vi "Create Map of Parameter Names.vi"(8 "error in (no error)":errorcluster, 11 "Kasli in":refnum<class "Kasli.lvclass">) -> (0 "error out":errorcluster, 2 "Parameters Map":map{string, string[]}(c390), 3 "Kasli out":refnum<class "Kasli.lvclass">)   [LabVIEW 2020, in "Kasli Wrapper 2.0.lvlib" / "Kasli.lvclass"]
doc: "This VI reads the Build and Init.py library and retrieves the mapping of Kasli names to the list of parameters for the script"
uses:
  Kasli.lvclass
  Kasli.lvclass/Kasli.ctl
  <vilib>/regexp/Match Regular Expression.xnode
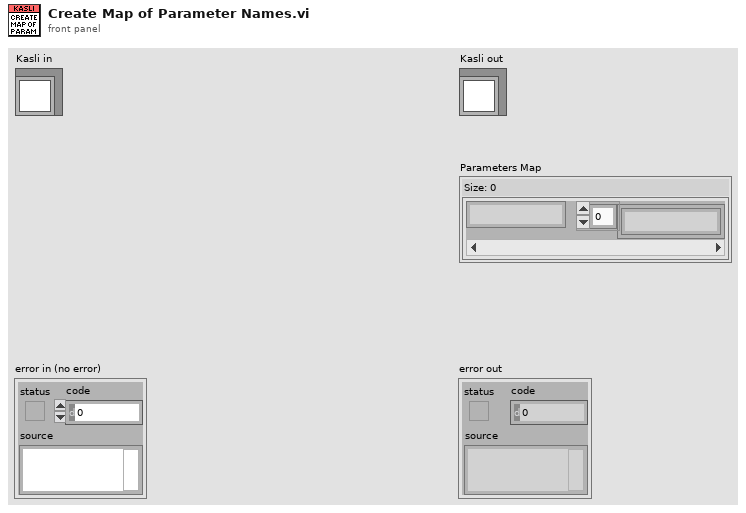
[diagram p1: front panel]
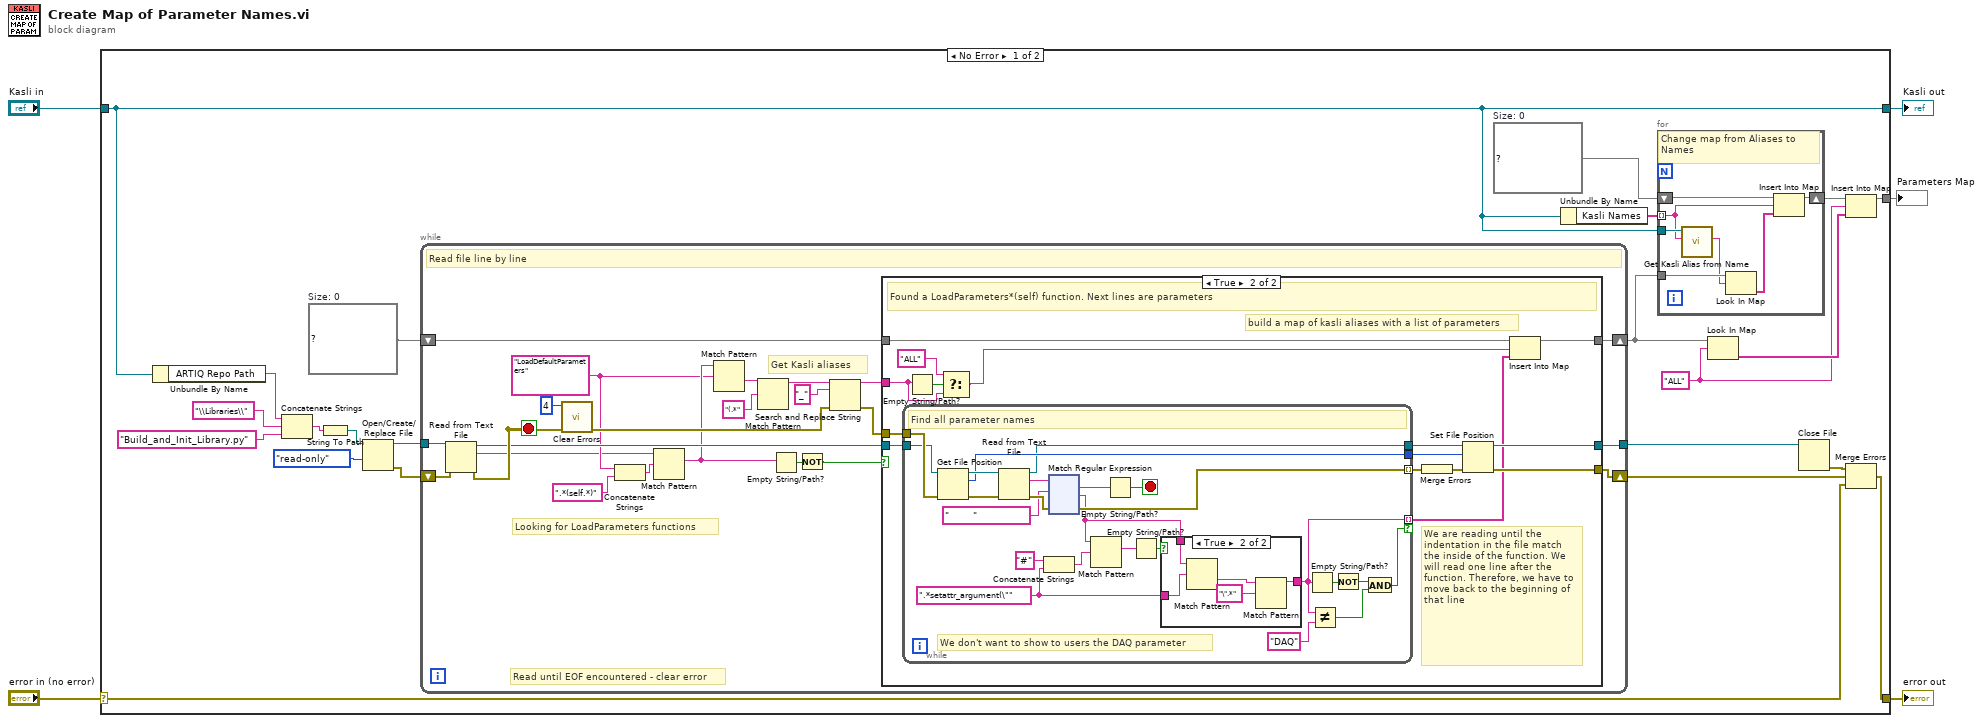
[diagram p0: block diagram]
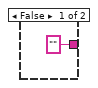
[diagram p3: hidden frame]
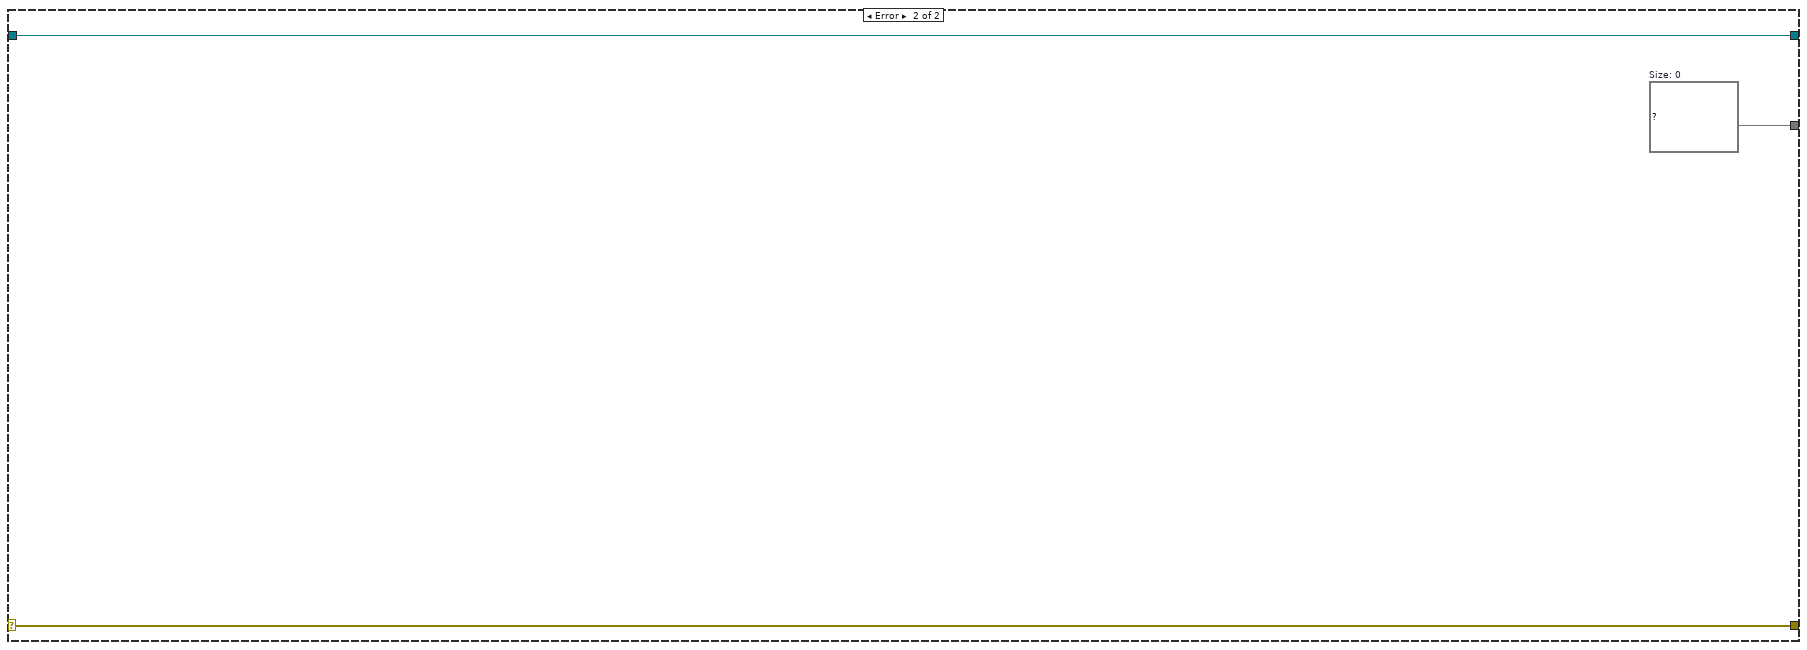
[diagram p4: hidden frame]
diagram:
  n1 = case shown="No Error" "error in (no error)" {
    selector: "error in (no error)" -> [w14 w222]
    tunnel: [w13 w222] -> w4
    tunnel: [w10 w221] -> w2
    tunnel: "Kasli in" -> [w10 w221]
    tunnel: [w9 w220] -> w1
    frame No Error {
      w6 = "ALL" ("key")
      w11 = map{string, string[]} {}  # Size: 0
      w23 = map{string, string[]} {}  # Size: 0
      n2 = Unbundle By Name(w10) -> ("ARTIQ Repo Path"=w16:string)
      n3 = Concatenate Strings(w16, "\\Libraries\\" ("string"), "Build_and_Init_Library.py") -> (w19:string)
      n4 = String To Path(string=w19) -> (path=w18:path)
      n5 = Open/Create/Replace File(file path (use dialog)=w18, access (0:read/write)=enum16{"read/write", "read-only", "write-only"}."read-only") -> (refnum out=w26:refnum<file>, error out=w15:errorcluster)  [unwired: 4 in, 1 out]
      n6 = while {
        tunnel: w26 -> [w55]
        tunnel: [w42] -> w25
        shift-right: [w46] -> w7
        shift-left: w23 -> [w47]
        shift-right: [w36] -> w22
        shift-left: w15 -> [w54]
        stop <- w56 stop-if-true
        w40 = "LoadDefaultParameters" ("regular expression")
        # "Get Kasli aliases"
        # "Looking for LoadParameters functions"
        # "Read until EOF encountered - clear error"
        # "Read file line by line"
        n7 = Read from Text File(file (use dialog)=w55, error in=w54) -> (refnum out=w44:refnum<file>, text=w35:string, error out=w56:errorcluster)  [unwired: 2 in, 1 out]
        n8 = call <vilib>:"Clear Errors.vi"("error in (no error)"=w56, "specific error code to clear (0: all)"=4) -> ("error out"=w57:errorcluster)  [unwired: 4 in, 1 out]
        n9 = Concatenate Strings(w40, ".*(self.*)" ("regular expression")) -> (w50:string)
        n10 = Match Pattern(string=w35, regular expression=w50) -> (match substring=w41:string)  [unwired: 1 in, 3 out]
        n11 = Match Pattern(string=w41, regular expression=w40) -> (after substring=w39:string)  [unwired: 1 in, 3 out]
        n12 = Match Pattern(string=w39, regular expression="(.*") -> (before substring=w37:string)  [unwired: 1 in, 3 out]
        n13 = Empty String/Path?(string/path=w41) -> (empty?=w52:bool)
        n14 = Not(x=w52) -> (.not. x?=w48:bool)
        n15 = Search and Replace String(input string=w37, search string="_", error in=w57) -> (result string=w45:string, error out=w43:errorcluster)  [unwired: 5 in, 2 out]
        n16 = case shown="True" w48 {
          tunnel: w47 -> [w60 w69]
          tunnel: [w60 w70] -> w46
          tunnel: w45 -> [_ w62]
          tunnel: w44 -> [w59 w75]
          tunnel: w43 -> [w58 w74]
          tunnel: [w59 w71] -> w42
          tunnel: [w58 w66] -> w36
          frame False {
            # "This line doesn't contain the LoadDefaultParamters function"
          }
          frame True {
            # "We are reading until the indentation in the file match the inside of the function. We will read one line after the function. Therefore, we have to move back to the beginning of that line"
            # "build a map of kasli aliases with a list of parameters"
            # "Found a LoadParameters*(self) function. Next lines are parameters"
            n17 = while {
              tunnel: w75 -> [w92]
              tunnel: w74 -> [w99]
              tunnel: [w80] -> w65 mode=indexing if=w76
              tunnel: [w87] -> w72
              tunnel: [w98] -> w67 mode=indexing
              tunnel: [w89] -> w73
              stop <- w93 stop-if-true
              w82 = ".*setattr_argument(\""
              # "We don't want to show to users the DAQ parameter"
              # "Find all parameter names"
              n18 = Get File Position(4:w99, 7:w92) -> (0:w90:errorcluster, 2:w89:i64, 3:w91:refnum<file>)
              n19 = Read from Text File(file (use dialog)=w91, error in=w90) -> (refnum out=w87:refnum<file>, text=w96:string, error out=w97:errorcluster)  [unwired: 2 in, 1 out]
              n20 = Concatenate Strings("#" ("string"), w82) -> (w83:string)
              n21 = xnode "Match Regular Expression"("input string"=w96, "regular expression"="        ", "error in"=w97) -> ("whole match"=w94:string, "after match"=w86:string, "error out"=w98:errorcluster)  [unwired: 3 in, 2 out]
              n22 = Match Pattern(string=w86, regular expression=w83) -> (match substring=w84:string)  [unwired: 1 in, 3 out]
              n23 = Empty String/Path?(string/path=w94) -> (empty?=w93:bool)
              n24 = Empty String/Path?(string/path=w84) -> (empty?=w85:bool)
              n25 = case shown="True" w85 {
                tunnel: ["" ("after match") w104] -> w80
                tunnel: w86 -> [_ w102]
                tunnel: w82 -> [_ w101]
                frame False {
                }
                frame True {
                  n26 = Match Pattern(string=w102, regular expression=w101) -> (after substring=w103:string)  [unwired: 1 in, 3 out]
                  n27 = Match Pattern(string=w103, regular expression="\".*" ("search string")) -> (before substring=w104:string)  [unwired: 1 in, 3 out]
                }
              }
              n28 = Empty String/Path?(string/path=w80) -> (empty?=w88:bool)
              n29 = Not Equal?(x=w80, y="DAQ") -> (x != y?=w77:bool)
              n30 = Not(x=w88) -> (.not. x?=w78:bool)
              n31 = And(x=w78, y=w77) -> (x .and. y?=w76:bool)
            }
            n32 = Empty String/Path?(string/path=w62) -> (empty?=w64:bool)
            n33 = Select(t="ALL", s=w64, f=w62) -> (s? t:f=w63:string)
            n34 = Merge Errors(w67) -> (w68:errorcluster)
            n35 = Set File Position(offset (in bytes) (0)=w73, refnum=w72, error in=w68) -> (refnum out=w71:refnum<file>, error out=w66:errorcluster)  [unwired: 1 in]
            n36 = Insert Into Map(map in=w69, key=w63, value=w65) -> (map out=w70:map{string, string[]})  [unwired: 2 out]
          }
        }
      }
      n37 = Unbundle By Name(w10) -> ("Kasli Names"=w12:string[])
      n38 = for {
        tunnel: w12 -> [w30] mode=indexing
        shift-right: [w33] -> w8
        shift-left: w11 -> [w34]
        tunnel: w7 -> [w32]
        tunnel: w10 -> [w31]
        # "Change map from Aliases to Names"
        n39 = call-dynamic "Get Kasli Alias from Name.vi"("Kasli Name"=w30, "Kasli in"=w31) -> ("Kasli Alias"=w29:string)  [unwired: 7 in, 2 out]
        n40 = Look In Map(map=w32, key=w29) -> (value=w28:string[])  [unwired: 1 in, 1 out]
        n41 = Insert Into Map(map in=w34, key=w30, value=w28) -> (map out=w33:map{string, string[]})  [unwired: 2 out]
      }
      n42 = Look In Map(map=w7, key=w6) -> (value=w27:string[])  [unwired: 1 in, 1 out]
      n43 = Close File(refnum=w25) -> (error out=w21:errorcluster)  [unwired: 1 in, 1 out]
      n44 = Insert Into Map(map in=w8, key=w6, value=w27) -> (map out=w9:map{string, string[]})  [unwired: 2 out]
      n45 = Merge Errors(w21, w22, w14) -> (w13:errorcluster)
    }
    frame Error {
      w220 = map{string, string[]} {}  # Size: 0
    }
  }
  "error out" <- w4
  "Kasli out" <- w2
  "Parameters Map" <- w1
